vi "UTILITY Initialize Front Panel Controls.vi"(11 "Initial DOE Config":path=path "C:/GE/Washer DOE 6") -> (3 "Initial DOE Config 2":path, 6 "Front Panel Controls DOE":T1)   [LabVIEW 2018]
uses:
  Washer DOE/Type Definitions/DOE Front Panel Controls.ctl
  <vilib>/Utility/error.llb/whitespace.ctl
  <vilib>/Utility/file.llb/Read From Spreadsheet File (string).vi
panel:
  out "file or folder exists?":bool
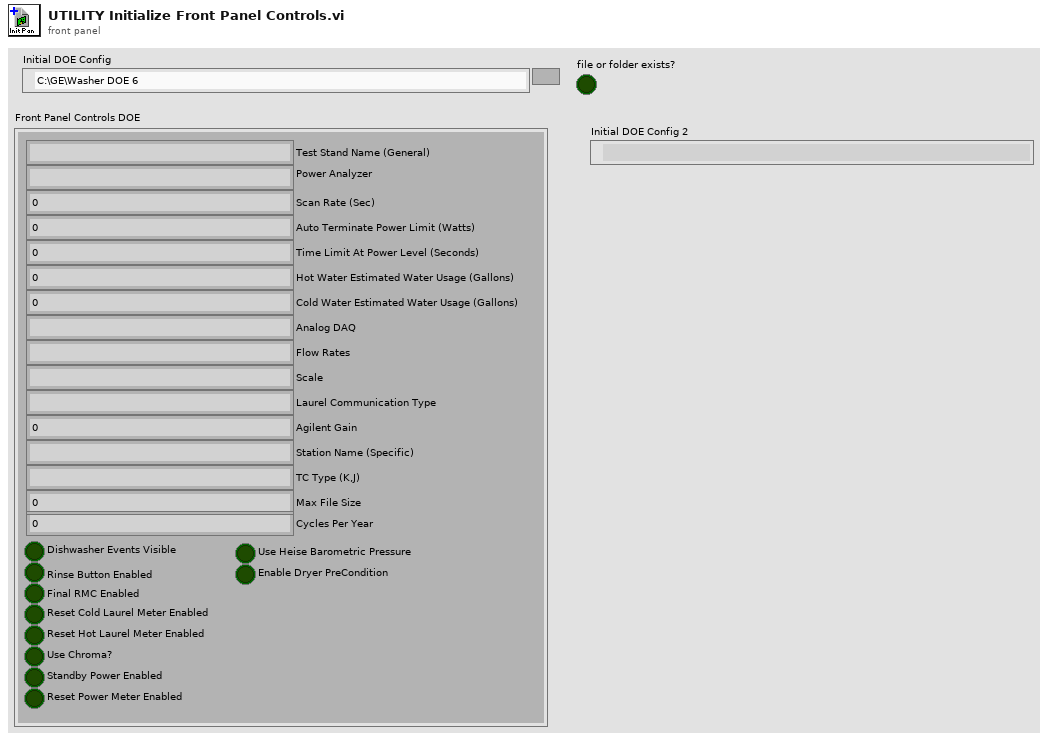
[diagram p1: front panel]
types:
  T1 = typedef "DOE Front Panel Controls.ctl" = cluster{"Test Stand Name (General)":string, "Power Analyzer":string, "Scan Rate (Sec)":dbl, "Auto Terminate Power Limit (Watts)":dbl, "Time Limit At Power Level (Seconds)":dbl, "Hot Water Estimated Water Usage (Gallons)":dbl, "Cold Water Estimated Water Usage (Gallons)":dbl, "Analog DAQ":string, "Flow Rates":string, "Scale":string, "Dishwasher Events Visible":bool, "Rinse Button Enabled":bool, "Final RMC Enabled":bool, "Reset Cold Laurel Meter Enabled":bool, "Laurel Communication Type":string, "Agilent Gain":dbl, "Station Name (Specific)":string, "TC Type (K,J)":string, "Max File Size":dbl, "Reset Hot Laurel Meter Enabled":bool, "Use Chroma?":bool, "Standby Power Enabled":bool, "Reset Power Meter Enabled":bool, "Use Heise Barometric Pressure":bool, "Enable Dryer PreCondition":bool, "Cycles Per Year":u32}
  T2 = typedef "whitespace.ctl" = u16
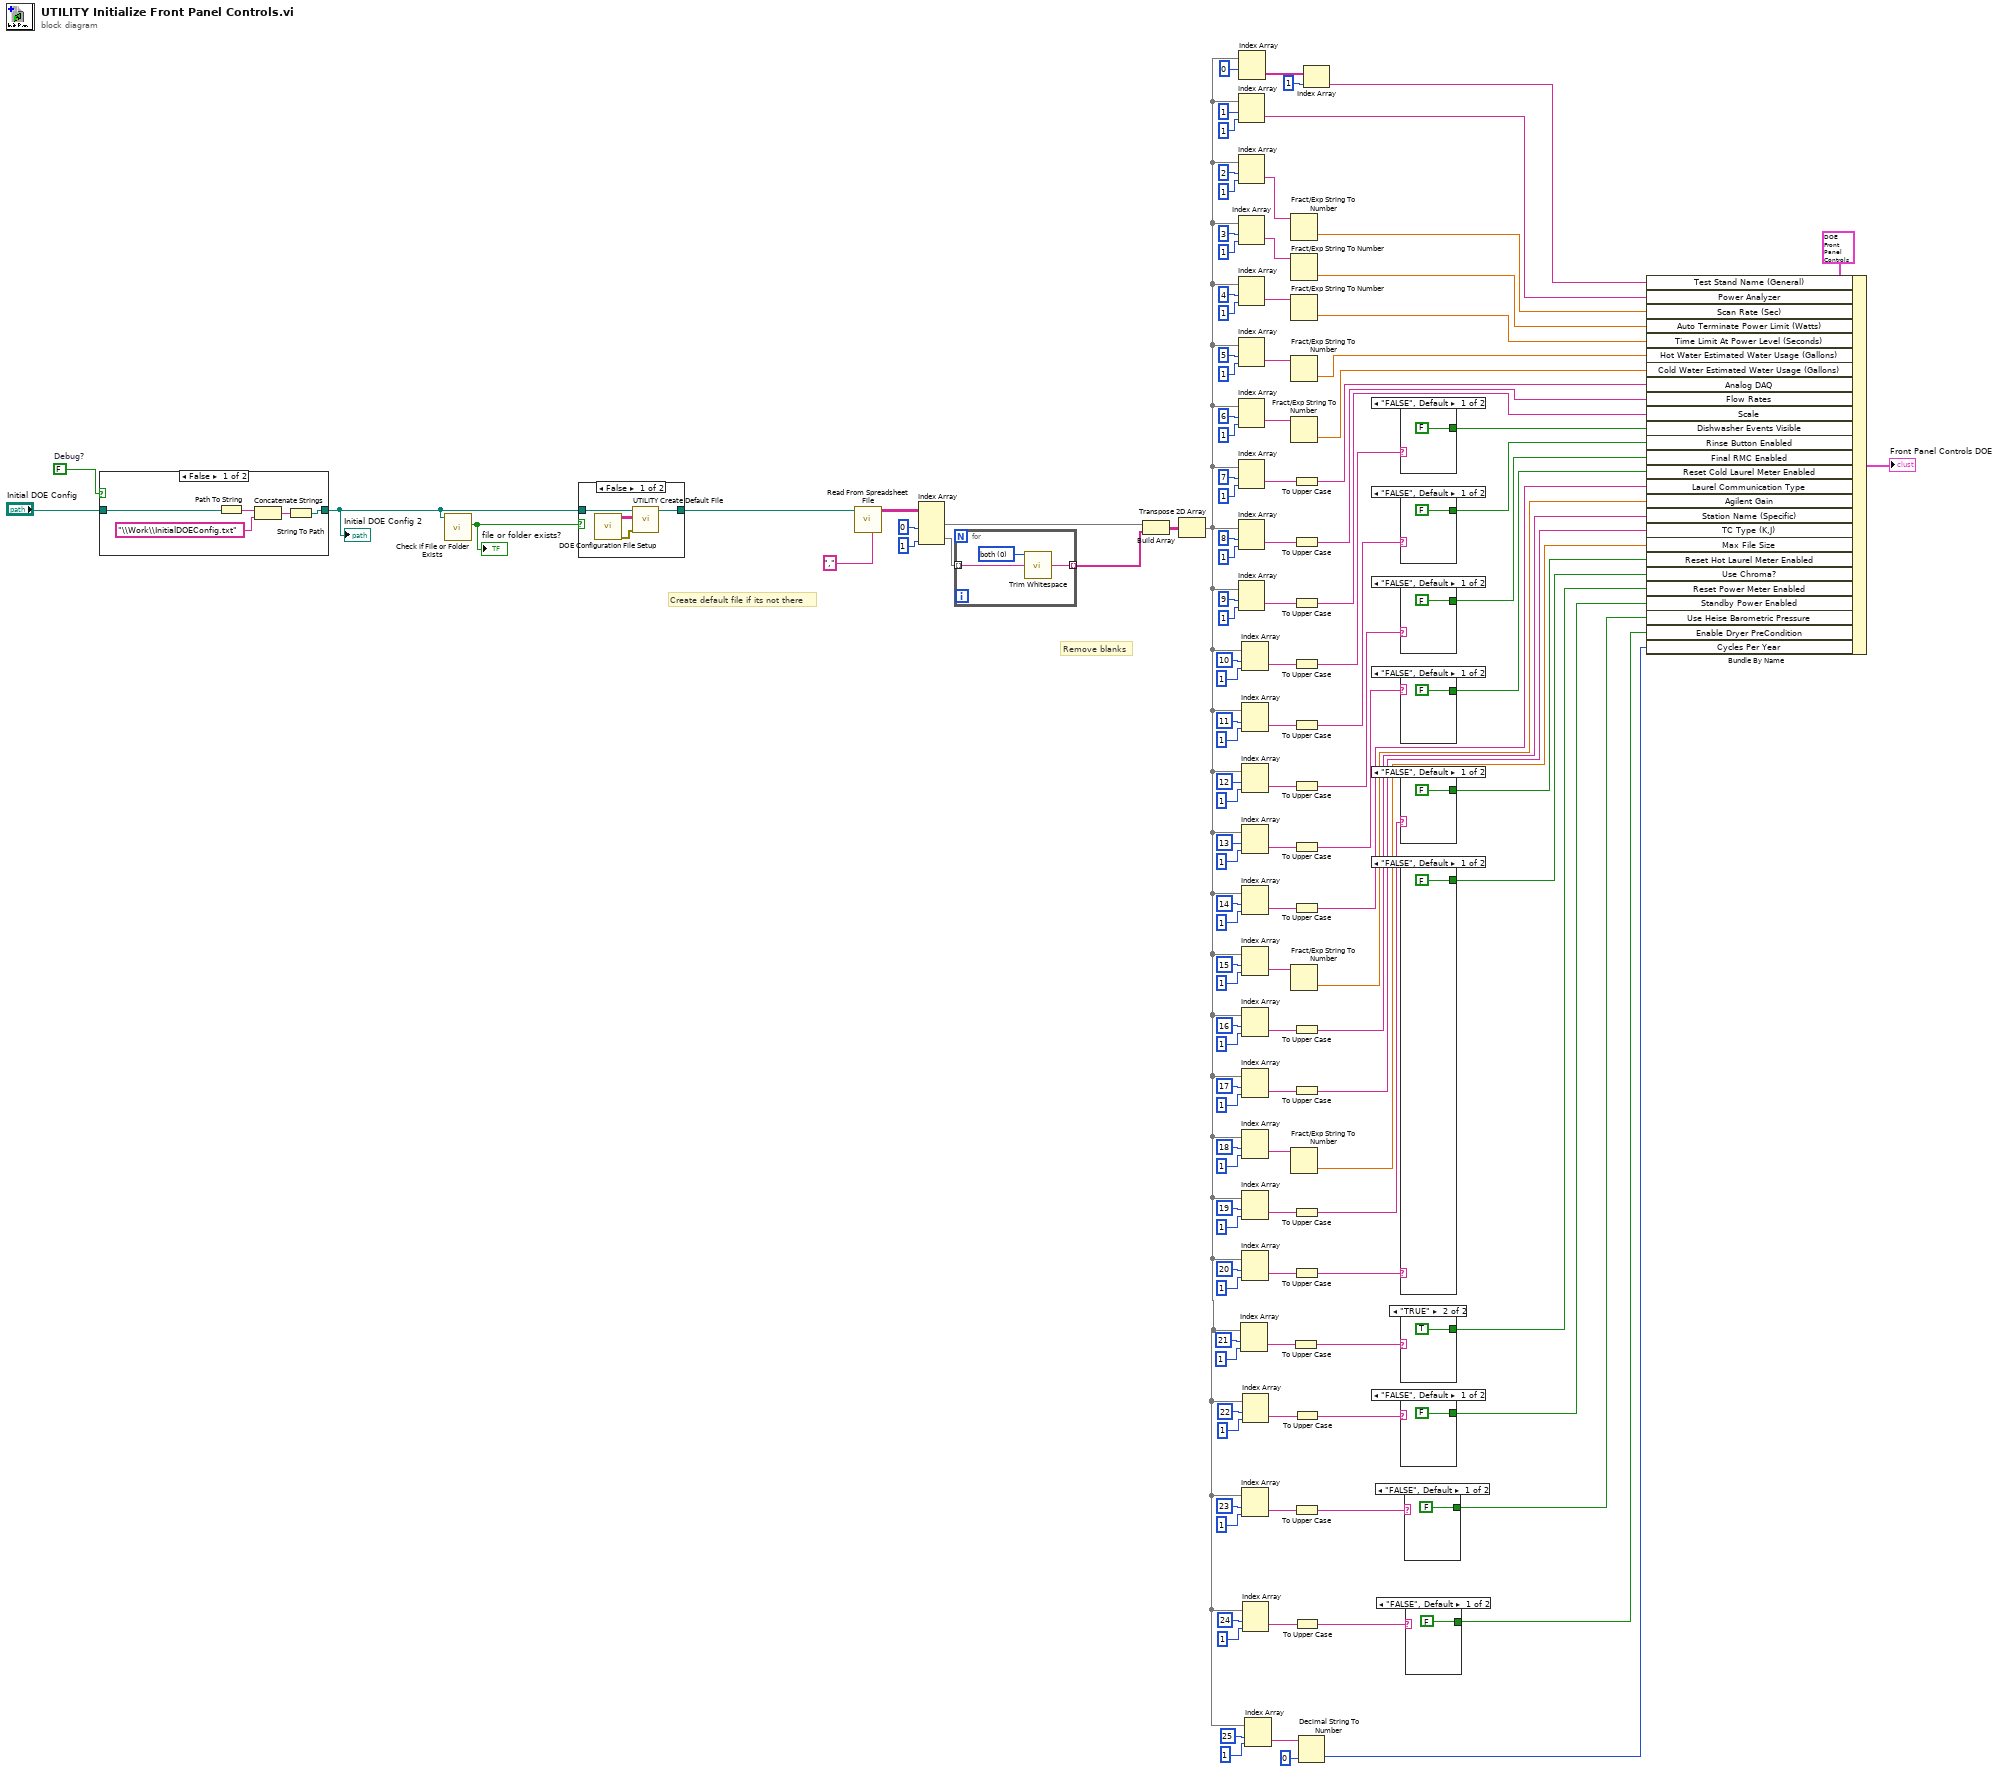
[diagram p0: block diagram]
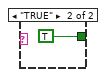
[diagram p2: hidden frame]
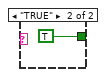
[diagram p3: hidden frame]
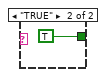
[diagram p4: hidden frame]
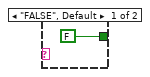
[diagram p5: hidden frame]
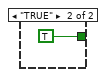
[diagram p6: hidden frame]
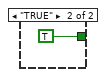
[diagram p7: hidden frame]
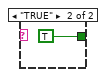
[diagram p9: hidden frame]
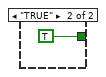
[diagram p10: hidden frame]
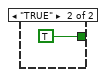
[diagram p11: hidden frame]
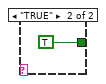
[diagram p12: hidden frame]
diagram:
  w50 = FALSE  # Debug?
  # "Remove blanks"
  # "Create default file if its not there"
  n1 = case shown="False" w50 {
    tunnel: "Initial DOE Config" -> [w135 w136]
    tunnel: [w131 w136] -> w42
    frame False {
      n2 = Path To String(path=w135) -> (string=w134:string)
      n3 = Concatenate Strings(w134, "\\Work\\InitialDOEConfig.txt") -> (w132:string)
      n4 = String To Path(string=w132) -> (path=w131:path)
    }
    frame True {
    }
  }
  "Initial DOE Config 2" <- w42
  n5 = call <vilib>:"Check if File or Folder Exists.vi"("path"=w42) -> ("file or folder exists?"=w108:bool)  [unwired: 8 in, 2 out]
  "file or folder exists?" <- w108
  n6 = case shown="False" w108 {
    tunnel: w42 -> [w140 w141]
    tunnel: [w139 w141] -> w107
    frame False {
      n7 = call "DOE Configuration File Setup.vi"() -> ("Error Out"=w138:errorcluster, "Config File"=w137:string[][])  [unwired: 10 in]
      n8 = call "UTILITY Create Default File.vi"("Error In"=w138, "Default File"=w137, "Initial DOE Config"=w140) -> ("new file path (Not A Path if cancelled)"=w139:path)  [unwired: 7 in, 1 out]
    }
    frame True {
    }
  }
  n9 = call-poly <vilib>:"Read From Spreadsheet File.vi"("delimiter (\\t)"="," ("delimiter (\\t)"), "file path (dialog if empty)"=w107) -> ("all rows"=w43:string[][])  [unwired: 5 in, 4 out]
  n10 = Index Array(array=w43, index (col) #1=0 ("disabled index (col)"), index (col) #2=1 ("disabled index (col)")) -> (element #1=w45:string[], element #2=w47:string[])  [unwired: 2 in]
  n11 = for {
    tunnel: w47 -> [w144] mode=indexing
    tunnel: [w142] -> w46 mode=indexing
    w143 = T2 0 items=["both", "start of string", "end of string"] ("location (both)")
    n12 = call <vilib>:"Trim Whitespace.vi"("string"=w144, "location (both)"=w143) -> ("trimmed string"=w142:string)
  }
  n13 = Build Array(w45, w46) -> (w44:string[][])
  n14 = Transpose 2D Array(2D array=w44) -> (transposed array=w5:string[][])
  n15 = Index Array(array=w5, index (row)=1 ("disabled index (row)"), index (col)=1 ("disabled index (col)")) -> (element=w122:string)
  n16 = Index Array(array=w5, index (row)=2 ("disabled index (row)"), index (col)=1 ("disabled index (col)")) -> (element=w117:string)
  n17 = Index Array(array=w5, index (row)=3 ("disabled index (row)"), index (col)=1 ("disabled index (col)")) -> (element=w116:string)
  n18 = Index Array(array=w5, index (row)=4 ("disabled index (row)"), index (col)=1 ("disabled index (col)")) -> (element=w115:string)
  n19 = Index Array(array=w5, index (row)=5 ("disabled index (row)"), index (col)=1 ("disabled index (col)")) -> (element=w101:string)
  n20 = Index Array(array=w5, index (row)=6 ("disabled index (row)"), index (col)=1 ("disabled index (col)")) -> (element=w102:string)
  n21 = Index Array(array=w5, index (row)=7 ("disabled index (row)"), index (col)=1 ("disabled index (col)")) -> (element=w68:string)
  n22 = Index Array(array=w5, index (row)=8 ("disabled index (row)"), index (col)=1 ("disabled index (col)")) -> (element=w67:string)
  n23 = Index Array(array=w5, index (row)=9 ("disabled index (row)"), index (col)=1 ("disabled index (col)")) -> (element=w65:string)
  n24 = Index Array(array=w5, index (row)=0) -> (element=w127:string[])  [unwired: 1 in]
  n25 = Index Array(array=w5, index (row)=21 ("disabled index (row)"), index (col)=1 ("disabled index (col)")) -> (element=w27:string)
  n26 = Index Array(array=w5, index (row)=10 ("disabled index (row)"), index (col)=1 ("disabled index (col)")) -> (element=w83:string)
  n27 = Index Array(array=w5, index (row)=11 ("disabled index (row)"), index (col)=1 ("disabled index (col)")) -> (element=w78:string)
  n28 = Index Array(array=w5, index (row)=12 ("disabled index (row)"), index (col)=1 ("disabled index (col)")) -> (element=w77:string)
  n29 = Index Array(array=w5, index (row)=13 ("disabled index (row)"), index (col)=1 ("disabled index (col)")) -> (element=w76:string)
  n30 = Index Array(array=w5, index (row)=14 ("disabled index (row)"), index (col)=1 ("disabled index (col)")) -> (element=w72:string)
  n31 = Index Array(array=w5, index (row)=15 ("disabled index (row)"), index (col)=1 ("disabled index (col)")) -> (element=w63:string)
  n32 = Index Array(array=w5, index (row)=16 ("disabled index (row)"), index (col)=1 ("disabled index (col)")) -> (element=w56:string)
  n33 = Index Array(array=w5, index (row)=17 ("disabled index (row)"), index (col)=1 ("disabled index (col)")) -> (element=w54:string)
  n34 = Index Array(array=w5, index (row)=18 ("disabled index (row)"), index (col)=1 ("disabled index (col)")) -> (element=w39:string)
  n35 = Index Array(array=w5, index (row)=19 ("disabled index (row)"), index (col)=1 ("disabled index (col)")) -> (element=w37:string)
  n36 = Index Array(array=w5, index (row)=20 ("disabled index (row)"), index (col)=1 ("disabled index (col)")) -> (element=w30:string)
  n37 = Index Array(array=w5, index (row)=23 ("disabled index (row)"), index (col)=1 ("disabled index (col)")) -> (element=w16:string)
  n38 = Index Array(array=w5, index (row)=22 ("disabled index (row)"), index (col)=1 ("disabled index (col)")) -> (element=w22:string)
  n39 = Index Array(array=w5, index (row)=24 ("disabled index (row)"), index (col)=1 ("disabled index (col)")) -> (element=w10:string)
  n40 = Index Array(array=w5, index (row)=25 ("disabled index (row)"), index (col)=1 ("disabled index (col)")) -> (element=w4:string)
  n41 = Fract/Exp String To Number(string=w117) -> (number=w112:dbl)  [unwired: 3 in, 1 out]
  n42 = Fract/Exp String To Number(string=w116) -> (number=w111:dbl)  [unwired: 3 in, 1 out]
  n43 = Fract/Exp String To Number(string=w115) -> (number=w110:dbl)  [unwired: 3 in, 1 out]
  n44 = Fract/Exp String To Number(string=w101) -> (number=w100:dbl)  [unwired: 3 in, 1 out]
  n45 = Fract/Exp String To Number(string=w102) -> (number=w99:dbl)  [unwired: 3 in, 1 out]
  n46 = Fract/Exp String To Number(string=w63) -> (number=w60:dbl)  [unwired: 3 in, 1 out]
  n47 = Fract/Exp String To Number(string=w39) -> (number=w38:dbl)  [unwired: 3 in, 1 out]
  n48 = To Upper Case(1:w27) -> (0:w21:string)
  n49 = To Upper Case(1:w68) -> (0:w1:string)
  n50 = To Upper Case(1:w67) -> (0:w66:string)
  n51 = To Upper Case(1:w65) -> (0:w64:string)
  n52 = To Upper Case(1:w83) -> (0:w82:string)
  n53 = To Upper Case(1:w78) -> (0:w81:string)
  n54 = To Upper Case(1:w77) -> (0:w80:string)
  n55 = To Upper Case(1:w76) -> (0:w79:string)
  n56 = To Upper Case(1:w72) -> (0:w69:string)
  n57 = To Upper Case(1:w56) -> (0:w55:string)
  n58 = To Upper Case(1:w54) -> (0:w51:string)
  n59 = To Upper Case(1:w37) -> (0:w34:string)
  n60 = To Upper Case(1:w30) -> (0:w29:string)
  n61 = To Upper Case(1:w16) -> (0:w17:string)
  n62 = To Upper Case(1:w22) -> (0:w20:string)
  n63 = To Upper Case(1:w10) -> (0:w9:string)
  n64 = Decimal String To Number(string=w4, default (0L)=u32 0 ("default (0 I32)")) -> (number=w3:u32)  [unwired: 1 in, 1 out]
  n65 = Index Array(array=w127, index=1) -> (element=w109:string)
  n66 = case shown="\"FALSE\", Default" w82 {
    tunnel: [FALSE TRUE] -> w84
    frame "FALSE", Default {
    }
    frame "TRUE" {
    }
  }
  n67 = case shown="\"FALSE\", Default" w81 {
    tunnel: [FALSE TRUE] -> w75
    frame "FALSE", Default {
    }
    frame "TRUE" {
    }
  }
  n68 = case shown="\"FALSE\", Default" w80 {
    tunnel: [FALSE TRUE] -> w74
    frame "FALSE", Default {
    }
    frame "TRUE" {
    }
  }
  n69 = case shown="\"FALSE\", Default" w79 {
    tunnel: [FALSE TRUE] -> w73
    frame "FALSE", Default {
    }
    frame "TRUE" {
    }
  }
  n70 = case shown="\"FALSE\", Default" w34 {
    tunnel: [FALSE TRUE] -> w33
    frame "FALSE", Default {
    }
    frame "TRUE" {
    }
  }
  n71 = case shown="\"FALSE\", Default" w29 {
    tunnel: [FALSE TRUE] -> w28
    frame "FALSE", Default {
    }
    frame "TRUE" {
    }
  }
  n72 = case shown="\"TRUE\"" w21 {
    tunnel: [FALSE TRUE] -> w19
    frame "FALSE", Default {
    }
    frame "TRUE" {
    }
  }
  n73 = case shown="\"FALSE\", Default" w20 {
    tunnel: [FALSE TRUE] -> w18
    frame "FALSE", Default {
    }
    frame "TRUE" {
    }
  }
  n74 = case shown="\"FALSE\", Default" w17 {
    tunnel: [FALSE TRUE] -> w13
    frame "FALSE", Default {
    }
    frame "TRUE" {
    }
  }
  n75 = case shown="\"FALSE\", Default" w9 {
    tunnel: [FALSE TRUE] -> w8
    frame "FALSE", Default {
    }
    frame "TRUE" {
    }
  }
  n76 = Bundle By Name(cluster=T1 {"Test Stand Name (General)"="", "Power Analyzer"="", "Scan Rate (Sec)"=0.0, "Auto Terminate Power Limit (Watts)"=0.0, "Time Limit At Power Level (Seconds)"=0.0, "Hot Water Estimated Water Usage (Gallons)"=0.0, "Cold Water Estimated Water Usage (Gallons)"=0.0, "Analog DAQ"="", "Flow Rates"="", "Scale"="", "Dishwasher Events Visible"=FALSE, "Rinse Button Enabled"=FALSE, "Final RMC Enabled"=FALSE, "Reset Cold Laurel Meter Enabled"=FALSE, "Laurel Communication Type"="", "Agilent Gain"=0.0, "Station Name (Specific)"="", "TC Type (K,J)"="", "Max File Size"=0.0, "Reset Hot Laurel Meter Enabled"=FALSE, "Use Chroma?"=FALSE, "Standby Power Enabled"=FALSE, "Reset Power Meter Enabled"=FALSE, "Use Heise Barometric Pressure"=FALSE, "Enable Dryer PreCondition"=FALSE, "Cycles Per Year"=0} ("Front Panel Controls DOE 2"), "Test Stand Name (General)"=w109, "Power Analyzer"=w122, "Scan Rate (Sec)"=w112, "Auto Terminate Power Limit (Watts)"=w111, "Time Limit At Power Level (Seconds)"=w110, "Hot Water Estimated Water Usage (Gallons)"=w100, "Cold Water Estimated Water Usage (Gallons)"=w99, "Analog DAQ"=w1, "Flow Rates"=w66, "Scale"=w64, "Dishwasher Events Visible"=w84, "Rinse Button Enabled"=w75, "Final RMC Enabled"=w74, "Reset Cold Laurel Meter Enabled"=w73, "Laurel Communication Type"=w69, "Agilent Gain"=w60, "Station Name (Specific)"=w55, "TC Type (K,J)"=w51, "Max File Size"=w38, "Reset Hot Laurel Meter Enabled"=w33, "Use Chroma?"=w28, "Reset Power Meter Enabled"=w19, "Standby Power Enabled"=w18, "Use Heise Barometric Pressure"=w13, "Enable Dryer PreCondition"=w8, "Cycles Per Year"=w3) -> (→"Front Panel Controls DOE":T1)
